vi "Initialize.vi"(8 "error in (no error)":errorcluster, 9 "Enqueuer ID string":string, 10 "Response Msg in":refnum<class "Response Msg.lvclass">, 11 "Response Core in":refnum<class "Interruptible Reply Core.lvclass">) -> (0 "error out":errorcluster, 1 "Wait for Response?":bool, 2 "Response Msg out":refnum<class "Response Msg.lvclass">, 3 "Response Core out":refnum<class "Interruptible Reply Core.lvclass">)   [LabVIEW 2020, in "Publisher.lvlib" / "Interruptible Reply Core.lvclass"]
doc: "Initialize the Response Core\n\nThis implementation obtains an interrupt notifier and a reply queue as well as registering the initialization time for timeout handling. \n\n'Wait for Response?' is set to TRUE."
uses:
  Interruptible Reply Core.lvclass
  Response Msg.lvclass
  Interruptible Reply Core.lvclass/Interruptible Reply Core.ctl
  PPL/HDH.Data.Generic.lvlibp/Synchronization/Notifier/Notifier.lvclass
  PPL/HDH.Data.Generic.lvlibp/Synchronization/Queue/Queue.lvclass
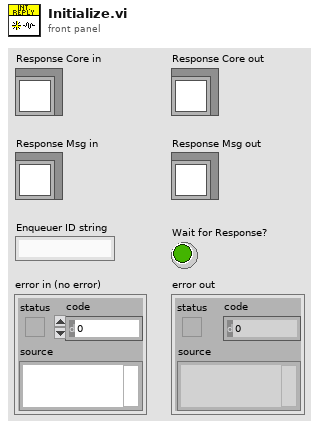
[diagram p1: front panel]
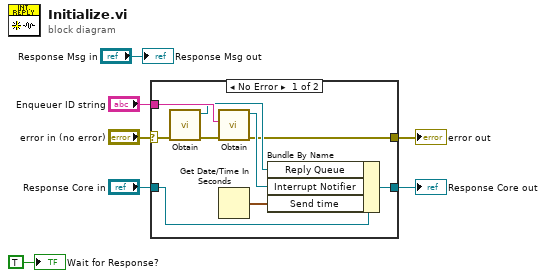
[diagram p0: block diagram]
diagram:
  n1 = case shown="No Error" "error in (no error)" {
    selector: "error in (no error)" -> [w13 w18]
    tunnel: "Enqueuer ID string" -> [w16 _]
    tunnel: [w9 w18] -> w2
    tunnel: "Response Core in" -> [w15 w17]
    tunnel: [w8 w17] -> w3
    frame No Error {
      n2 = call "Obtain.vi"("error in (no error)"=w13) -> ("error out"=w12:errorcluster, "Queue out"=w14:refnum<class "Queue.lvclass">)  [unwired: 8 in, 1 out]
      n3 = call "Obtain.vi"("error in (no error)"=w12, "Name (\"\")"=w16) -> ("error out"=w9:errorcluster, "Notifier out"=w10:refnum<class "Notifier.lvclass">)  [unwired: 7 in, 1 out]
      n4 = Get Date/Time In Seconds() -> (seconds since 1Jan1904=w11:timestamp)
      n5 = Bundle By Name(cluster=w15, "Reply Queue"=w14, "Interrupt Notifier"=w10, "Send time"=w11) -> (w8:refnum<class "Interruptible Reply Core.lvclass">)
    }
    frame Error {
    }
  }
  "error out" <- w2
  "Response Core out" <- w3
  "Response Msg out" <- "Response Msg in"
  "Wait for Response?" <- TRUE ("Wait for Response?")
